vi "Init Core.vi"(0 "Display State In":T2={"WebView2 Ref"=refnum, "event callback refnum"=refnum, "Events"={"Navigation Complete Event"=refnum, "Source Changed Event"=refnum, "Document Title Changed Event"=refnum, "Status Bar Text Changed"=refnum, "Web Message Received"=refnum, "Window Close Requested"=refnum}, "Paths"={"Webview2 Native"=path "C:/Users/kleins/Desktop/webview2/microsoft.web.webview2.1.0.1370.28/build/native", "Edge Application"=path "", "User Data"=path ""}}, 5 "Path Overrides":T1, 9 "Container State":T3, 11 "error in (no error)":errorcluster) -> (4 "Display State Out":T2={"WebView2 Ref"=refnum, "event callback refnum"=refnum, "Events"={"Navigation Complete Event"=refnum, "Source Changed Event"=refnum, "Document Title Changed Event"=refnum, "Status Bar Text Changed"=refnum, "Web Message Received"=refnum, "Window Close Requested"=refnum}, "Paths"={"Webview2 Native"=path "C:/Users/kleins/Desktop/webview2/microsoft.web.webview2.1.0.1370.28/build/native", "Edge Application"=path "", "User Data"=path ""}}, 15 "error out":errorcluster)   [LabVIEW 2020, in "WebView2 Control.xctl"]
uses:
  WebView2 Control.xctl
  <vilib>/_xctls/Container State.ctl
  State.ctl
  C:/Users/kleins/Desktop/webview2/microsoft.web.webview2.1.0.1370.28/lib/net45/Microsoft.Web.WebView2.WinForms.dll
  microsoft.web.webview2.1.0.1370.28/lib/net45/Microsoft.Web.WebView2.WinForms.dll
  Paths.ctl
  <vilib>/_xctls/XControlSupport.lvlib
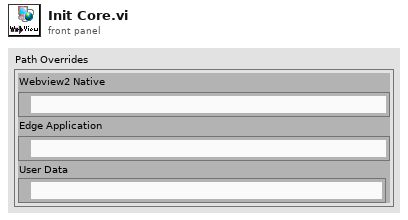
[diagram p1: front panel]
types:
  T1 = typedef "WebView2 Control.xctl/Paths.ctl" = cluster{"Webview2 Native":path, "Edge Application":path, "User Data":path}
  T2 = typedef "WebView2 Control.xctl/State.ctl" = cluster{"WebView2 Ref":refnum<data-value>, "event callback refnum":refnum<k27>, "Events":cluster{"Navigation Complete Event":refnum<user-event>, "Source Changed Event":refnum<user-event>, "Document Title Changed Event":refnum<user-event>, "Status Bar Text Changed":refnum<user-event>, "Web Message Received":refnum<user-event>, "Window Close Requested":refnum<user-event>}, "Paths":T1}
  T3 = typedef "XControlSupport.lvlib/Container State.ctl" = cluster{"Indicator?":bool, "Run Mode?":bool, " Refnum":refnum<vi>}
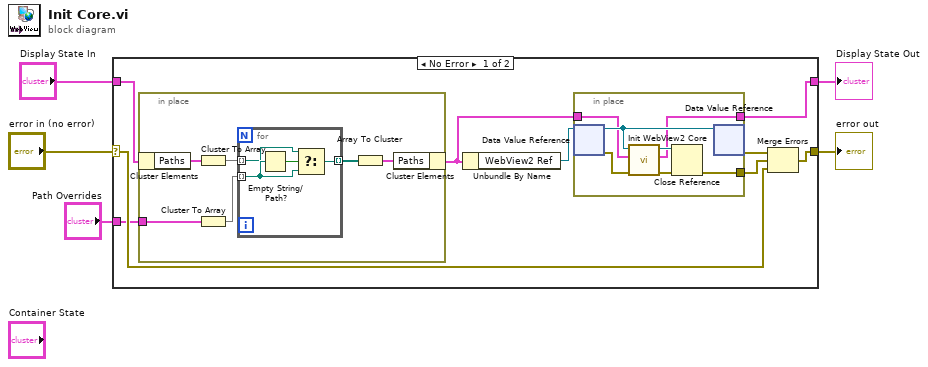
[diagram p0: block diagram]
diagram:
  n1 = case shown="No Error" "error in (no error)" {
    selector: "error in (no error)" -> [w14 w33]
    tunnel: "Display State In" -> [w12 w32]
    tunnel: [w11 w32] -> w3
    tunnel: [w10 w33] -> w2
    tunnel: "Path Overrides" -> [w6 _]
    frame No Error {
      n2 = in-place {
        in-place-border: w6 -> [w20]
        n3 = in-place-cluster #1(w12) -> ("Paths"=w19:T1)
        n4 = Cluster To Array(cluster=w19) -> (array=w18:path[])
        n5 = Cluster To Array(cluster=w20) -> (array=w15:path[])
        n6 = for {
          tunnel: [w24] -> w17 mode=indexing
          tunnel: w18 -> [w21] mode=indexing
          tunnel: w15 -> [w22] mode=indexing
          n7 = Empty String/Path?(string/path=w22) -> (empty?=w23:bool)
          n8 = Select(t=w21, s=w23, f=w22) -> (s? t:f=w24:path)
        }
        n9 = Array To Cluster(array=w17) -> (cluster=w16:cluster{"[0]":path, "[1]":path, "[2]":path})
        n10 = in-place-cluster #1("Paths"=w16) -> (w7:T2)
      }
      n11 = Unbundle By Name(w7) -> ("WebView2 Ref"=w13:refnum<data-value>)
      n12 = in-place {
        in-place-border: [w27] -> w11
        in-place-border: [w26] -> w9
        in-place-border: w7 -> [w25]
        n13 = in-place-dvr #2(w13) -> (w31:refnum<k24>, w28:errorcluster)
        n14 = call "Init WebView2 Core.vi"("error in (no error)"=w28, "Display State In"=w25, ".NET Refnum in"=w31) -> ("error out"=w29:errorcluster, "Display State In 2"=w27:T2, ".NET Refnum out"=w30:refnum<k24>)  [unwired: 6 in]
        n15 = Close Reference(reference=w30, error in (no error)=w29) -> (error out=w26:errorcluster)
        n16 = in-place-dvr #2(w31) -> (w8:errorcluster)  [unwired: 1 out]
      }
      n17 = Merge Errors(w8, w9, w14) -> (w10:errorcluster)
    }
    frame Error {
    }
  }
  "Display State Out" <- w3
  "error out" <- w2
